vi "Interface.vi"(8 "Error In":errorcluster) -> (0 "Error Out":errorcluster)   [LabVIEW 2018]
uses:
  UserInterface.lvlib
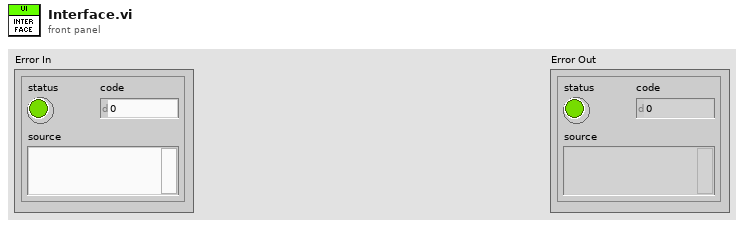
[diagram p1: front panel]
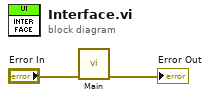
[diagram p0: block diagram]
diagram:
  n1 = call "Main.vi"("Error In"="Error In") -> ("Error Out"=→"Error Out":errorcluster)  [unwired: 10 in]
